vi "Add SPI Configuration.vi"(8 "error in (no error)":errorcluster, 10 "SPI Configuration in":refnum<k24>, 11 "Item Ref in":T1 format="%.0x") -> (0 "error out":errorcluster, 2 "SPI Configuration out":refnum<k24>, 3 "Item Ref out":T1 format="%.0x")   [LabVIEW 2014, in "SLSC configuration System Explorer.lvlib"]
uses:
  SLSC configuration System Explorer.lvlib
  C:/Files/Custom VeriStand Development/DET-SPI-Tool/XML Deserializer/SLSC Deserializer/SLSC Deserializer/bin/Release/SLSC Deserializer.dll
  XML Deserializer/SLSC Deserializer/SLSC Deserializer/bin/Release/SLSC Deserializer.dll
  <vilib>/NI Veristand/Custom Device API/Custom Device Item Ref.ctl
  <vilib>/NI Veristand/Custom Device API/Custom Device API.lvlib
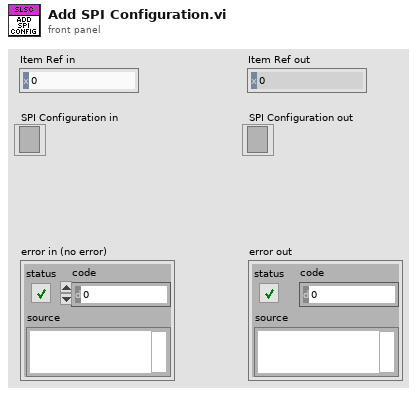
[diagram p1: front panel]
types:
  T1 = typedef "Custom Device API.lvlib/Custom Device Item Ref.ctl" = u64
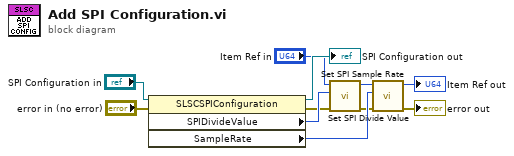
[diagram p0: block diagram]
diagram:
  n1 = property class="SLSCSPIConfiguration"(reference="SPI Configuration in", error in="error in (no error)") -> (reference out=→"SPI Configuration out":refnum<k24>, error out=w7:errorcluster, "SPIDivideValue"=w8:u16, "SampleRate"=w10:u32)
  n2 = call "Set SPI Divide Value.vi"("error in (no error)"=w7, "SPI Divide Value"=w8, "Item Ref in"="Item Ref in") -> ("error out"=w9:errorcluster, "Item Ref out"=w11:T1)  [unwired: 7 in]
  n3 = call "Set SPI Sample Rate.vi"("error in (no error)"=w9, "Sample Rate (S/s)"=w10, "Item Ref in"=w11) -> ("error out"=→"error out":errorcluster, "Item Ref out"=→"Item Ref out":T1)  [unwired: 7 in]
